vi "TempStabilitySettings.vi"() -> (1 "Diff Threshold":dbl, 2 "Short Time (2-secs)":dbl, 3 "Long Time (2-secs)":dbl)   [LabVIEW 2023]
panel:
  in  "OK Button":bool
  in  "Temerature Sensor":u16(ring)
  in  "Difference Threshold":dbl
  in  "Short Time (mins)":dbl
  in  "Long Time (mins)":dbl
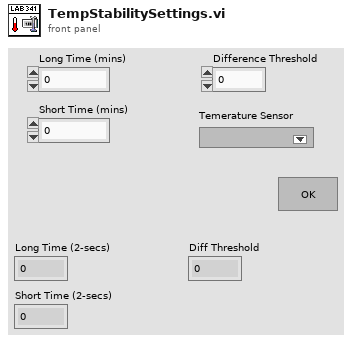
[diagram p1: front panel]
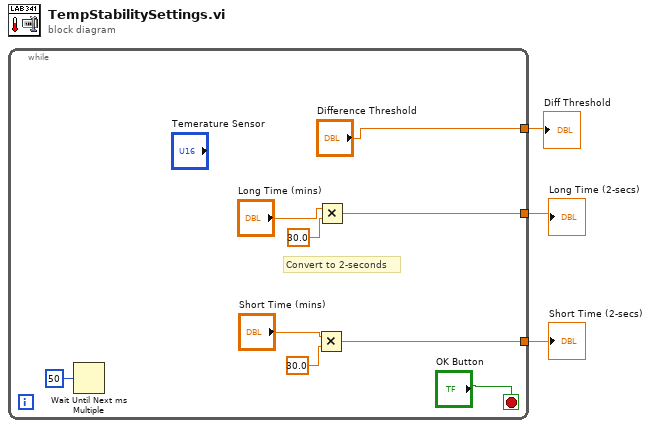
[diagram p0: block diagram]
diagram:
  n1 = while {
    tunnel: [w6] -> w3
    tunnel: ["Difference Threshold"] -> w2
    tunnel: [w4] -> w1
    stop <- "OK Button" stop-if-true
    # "Convert to 2-seconds"
    n2 = Wait Until Next ms Multiple(millisecond multiple=u32 50) -> ()  [unwired: 1 out]
    n3 = Multiply(x="Short Time (mins)", y=30.0 ("x")) -> (x*y=w4:dbl)
    n4 = Multiply(x="Long Time (mins)", y=30.0 ("x")) -> (x*y=w6:dbl)
  }
  "Diff Threshold" <- w2
  "Long Time (2-secs)" <- w3
  "Short Time (2-secs)" <- w1
